vi "Tclk parameters.vi"(8 "variant":variant, 9 "Options":T4={"GetInfo"=TRUE, "Set Det A para"=TRUE, "Set WD"=FALSE, "Set Mag"=TRUE, "Set stig"=FALSE, "Set aln"=FALSE, "Display"=TRUE, "Save"=TRUE, "8-bit"=TRUE, "Detector A"=TRUE, "Detector B"=TRUE, "Detector C"=FALSE, "Detector D"=FALSE, "Inverse A"=FALSE, "Inverse B"=FALSE, "Inverse C"=FALSE, "Inverse D"=FALSE, "Inverse PNG"=FALSE, "Freeze"=TRUE, "PNG only"=FALSE, "Upload"=TRUE, "Delete after upload"=FALSE}, 10 "Scan Para":T2={"X resolution"=0, "Y resolution"=0, "X center (um)"=0.0, "Y center (um)"=0.0, "X size (V)"=0.0, "X size auto"=TRUE, "X stig"=0.0, "Y stig"=0.0, "X aln"=0.0, "Y aln"=0.0, "Scan rate (Hz)"=0, "Oversampling"=0, "Oversampling auto"=TRUE, "Frame line rampdown ratio"=0.0, "Pixel size (nm)"=0.0, "WD"=0.0} {"WD" format="%#_7g"; "Frame line rampdown ratio" min=-1 max=1 step=0.05 format="%.2g"; "Scan rate (Hz)" max=4000000 format="%.2e"}, 11 "HW Config":T3={"SEM X coil"="", "SEM Y coil"="", "Detectors"="", "Det min (V)"=-10.0, "Det max (V)"=10.0, "Eanable COM"=TRUE, "COM port"="", "Detector FIB-NI auto switch"="", "Machine Type"=0, "Machine ID"="", "SEM Max FOV (um)"=350.0} {"Machine Type" items=["Feiss", "NVision"]}) -> (0 "Same tclk para?":bool, 3 "Tclk para out":T1={"SEM X coil"="", "SEM Y coil"="", "Detectors"="", "Det min (V)"=-10.0, "Det max (V)"=10.0, "X resolution"=0, "Y resolution"=0, "X size (V)"=0.0, "Scan rate (Hz)"=0, "Oversampling"=0, "Frame line rampdown ratio"=0.0, "Pixel size (nm)"=0.0, "Detector A"=TRUE, "Detector B"=TRUE, "Detector C"=FALSE, "Detector D"=FALSE} {"Frame line rampdown ratio" min=-1 max=1 step=0.05 format="%.2g"; "Scan rate (Hz)" max=4000000 format="%.2e"})   [LabVIEW 2018]
panel:
  # "Det"
  # "Det"
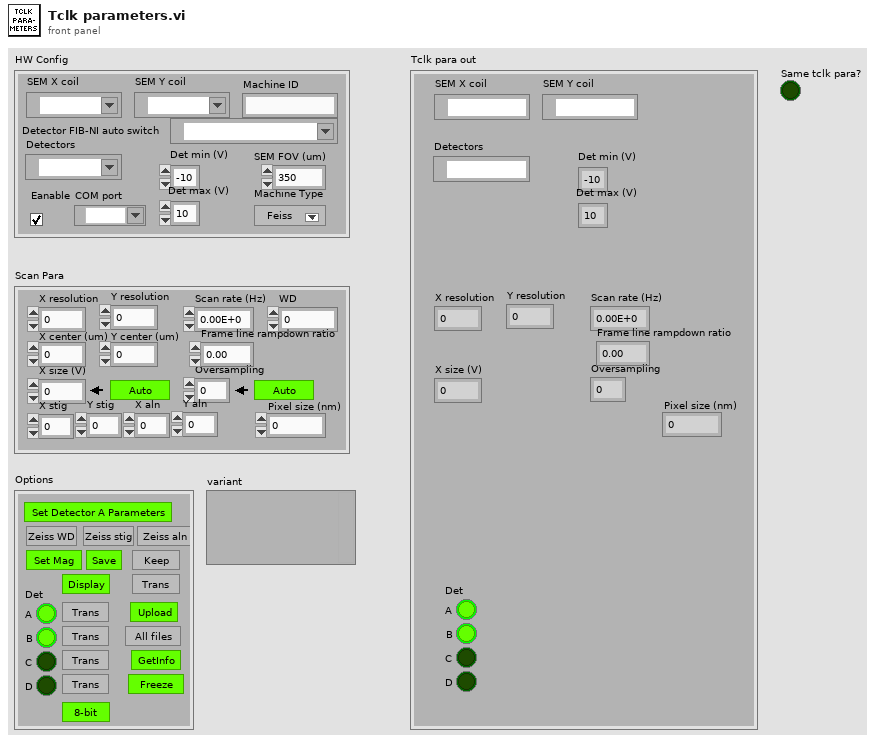
[diagram p1: front panel]
types:
  T1 = cluster{"SEM X coil":refnum<k15>, "SEM Y coil":refnum<k15>, "Detectors":refnum<k15>, "Det min (V)":sgl, "Det max (V)":sgl, "X resolution":u32, "Y resolution":u32, "X size (V)":sgl, "Scan rate (Hz)":u32, "Oversampling":u32, "Frame line rampdown ratio":sgl, "Pixel size (nm)":sgl, "Detector A":bool, "Detector B":bool, "Detector C":bool, "Detector D":bool}
  T2 = cluster{"X resolution":u32, "Y resolution":u32, "X center (um)":dbl, "Y center (um)":dbl, "X size (V)":dbl, "X size auto":bool, "X stig":sgl, "Y stig":sgl, "X aln":sgl, "Y aln":sgl, "Scan rate (Hz)":u32, "Oversampling":u32, "Oversampling auto":bool, "Frame line rampdown ratio":sgl, "Pixel size (nm)":sgl, "WD":sgl}
  T3 = cluster{"SEM X coil":refnum<k15>, "SEM Y coil":refnum<k15>, "Detectors":refnum<k15>, "Det min (V)":dbl, "Det max (V)":dbl, "Eanable COM":bool, "COM port":refnum<visa-resource-name>, "Detector FIB-NI auto switch":tag, "Machine Type":u8, "Machine ID":string, "SEM Max FOV (um)":sgl}
  T4 = cluster{"GetInfo":bool, "Set Det A para":bool, "Set WD":bool, "Set Mag":bool, "Set stig":bool, "Set aln":bool, "Display":bool, "Save":bool, "8-bit":bool, "Detector A":bool, "Detector B":bool, "Detector C":bool, "Detector D":bool, "Inverse A":bool, "Inverse B":bool, "Inverse C":bool, "Inverse D":bool, "Inverse PNG":bool, "Freeze":bool, "PNG only":bool, "Upload":bool, "Delete after upload":bool}
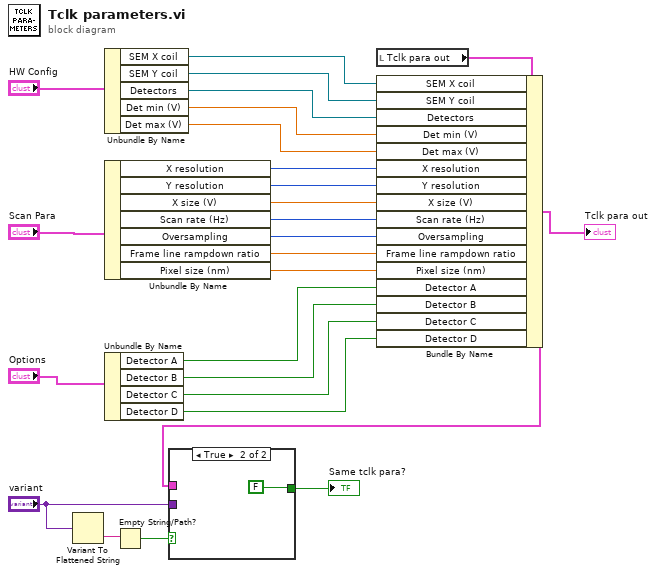
[diagram p0: block diagram]
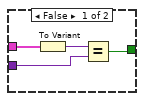
[diagram p2: hidden frame]
diagram:
  n1 = Variant To Flattened String(Variant="variant") -> (data string=w4:string)  [unwired: 1 out]
  n2 = Unbundle By Name("HW Config") -> ("SEM X coil"=w25:refnum<k15>, "SEM Y coil"=w24:refnum<k15>, "Detectors"=w23:refnum<k15>, "Det min (V)"=w22:dbl, "Det max (V)"=w21:dbl)
  n3 = Unbundle By Name("Scan Para") -> ("X resolution"=w20:u32, "Y resolution"=w19:u32, "X size (V)"=w18:dbl, "Scan rate (Hz)"=w17:u32, "Oversampling"=w16:u32, "Frame line rampdown ratio"=w15:sgl, "Pixel size (nm)"=w14:sgl)
  n4 = Unbundle By Name("Options") -> ("Detector A"=w13:bool, "Detector B"=w12:bool, "Detector C"=w11:bool, "Detector D"=w10:bool)
  n5 = Empty String/Path?(string/path=w4) -> (empty?=w3:bool)
  n6 = local read "Tclk para out"() -> (w5:T1)
  n7 = Bundle By Name(cluster=w5, "SEM X coil"=w25, "SEM Y coil"=w24, "Detectors"=w23, "Det min (V)"=w22, "Det max (V)"=w21, "X resolution"=w20, "Y resolution"=w19, "X size (V)"=w18, "Scan rate (Hz)"=w17, "Oversampling"=w16, "Frame line rampdown ratio"=w15, "Pixel size (nm)"=w14, "Detector A"=w13, "Detector B"=w12, "Detector C"=w11, "Detector D"=w10) -> (w1:T1)
  "Tclk para out" <- w1
  n8 = case shown="True" w3 {
    tunnel: [w26 FALSE] -> w6
    tunnel: "variant" -> [w27 _]
    tunnel: w1 -> [w29 _]
    frame False {
      n9 = To Variant(anything=w29) -> (Variant=w28:variant)
      n10 = Equal?(x=w28, y=w27) -> (x = y?=w26:bool)
    }
    frame True {
    }
  }
  "Same tclk para?" <- w6
